vi "Battery Switch States to Word.vi"(11 "Battery Switch States":T1) -> (3 "Battery Switch Word":u16)   [LabVIEW 2014, in "SLSC configuration Shared.lvlib"]
doc: "Converts four faults to a fault word."
uses:
  SLSC configuration Shared.lvlib
  Battery Switch Array.ctl
  Battery Switch.ctl
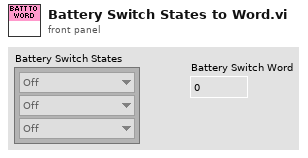
[diagram p1: front panel]
types:
  T1 = typedef "SLSC configuration Shared.lvlib/Battery Switch Array.ctl" = T2[]
  T2 = typedef "SLSC configuration Shared.lvlib/Battery Switch.ctl" = enum8{"Off", "On"}
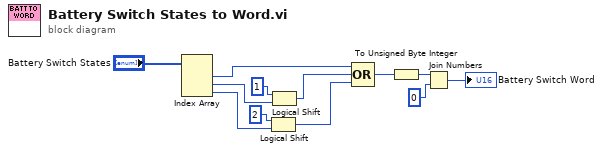
[diagram p0: block diagram]
diagram:
  n1 = Index Array(array="Battery Switch States") -> (element #1=w10:T2, element #2=w6:T2, element #3=w7:T2)  [unwired: 3 in]
  n2 = Logical Shift(y=u16 2, x=w7) -> (x << y=w12:u32)
  n3 = Logical Shift(y=u16 1, x=w6) -> (x << y=w11:u32)
  n4 = Compound Arithmetic op=OR(w10, w11, w12) -> (w4:u32)
  n5 = To Unsigned Byte Integer(number=w4) -> (unsigned 8bit integer=w1:u8)
  n6 = Join Numbers(hi=w1, lo=u8 0) -> ((hi.lo)=→"Battery Switch Word":u16)
